vi "Read Hardware Interface Information.vi"(8 "error in (no error)":errorcluster, 10 "hardware interface index":u16, 11 "PLBB in":refnum<class "PL BlackBox Modbus Client.lvclass">) -> (0 "error out":errorcluster, 2 "hardware interface information":cluster{"type":u16, "name":string} {"type" items=["Unknown", "UART", "Network interface", "Ethernet", "Wi-Fi"]}, 3 "PLBB out":refnum<class "PL BlackBox Modbus Client.lvclass">)   [LabVIEW 2015, in "PL BlackBox Modbus Client.lvclass"]
doc: "Reads the hardware interface information."
uses:
  PL BlackBox Modbus Client.lvclass
  <vilib>/plasmapper/PL Modbus Client/PL Modbus Client.lvclass
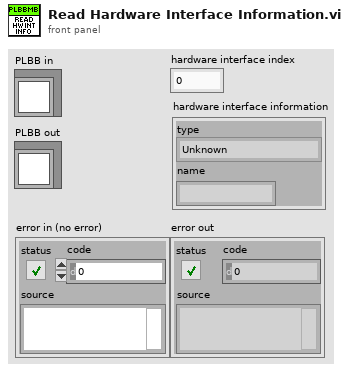
[diagram p1: front panel]
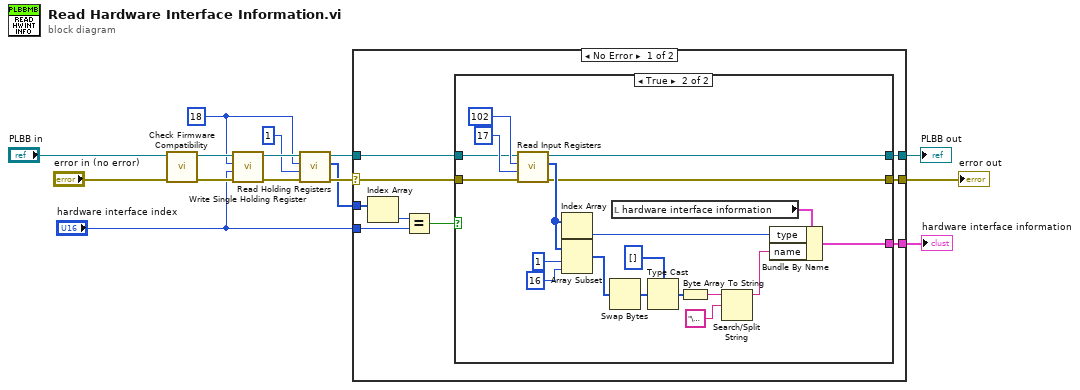
[diagram p0: block diagram]
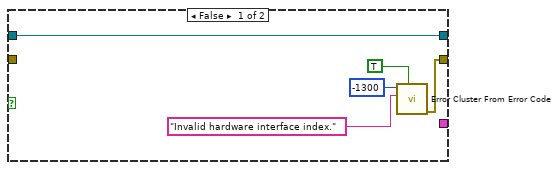
[diagram p2: hidden frame]
diagram:
  w7 = u16 18 ("address")
  n1 = call-dynamic "Check Firmware Compatibility.vi"("error in (no error)"="error in (no error)", "PLBB in"="PLBB in") -> ("error out"=w10:errorcluster, "PLBB out"=w11:refnum<class "PL BlackBox Modbus Client.lvclass">)  [unwired: 8 in]
  n2 = call <vilib>:"Write Single Holding Register.vi"("error in (no error)"=w10, "value"="hardware interface index", "address"=w7, "MODBUS in"=w11) -> ("error out"=w6:errorcluster, "MODBUS out"=w9:refnum<class "PL BlackBox Modbus Client.lvclass">)  [unwired: 6 in]
  n3 = call <vilib>:"Read Holding Registers.vi"("error in (no error)"=w6, "number of holding registers"=u16 1 ("address"), "address"=w7, "MODBUS in"=w9) -> ("error out"=w5:errorcluster, "values"=w3:u16[], "MODBUS out"=w4:refnum<class "PL BlackBox Modbus Client.lvclass">)  [unwired: 5 in]
  n4 = case shown="No Error" w5 {
    selector: w5 -> [w17 w49]
    tunnel: [w24 w49] -> w15
    tunnel: [w23 w50] -> w14
    tunnel: w4 -> [w18 w50]
    tunnel: w3 -> [w22 _]
    tunnel: "hardware interface index" -> [w20 _]
    tunnel: [w16 _] -> w1
    frame No Error {
      n5 = Index Array(array=w22) -> (element=w21:u16)  [unwired: 1 in]
      n6 = Equal?(x=w21, y=w20) -> (x = y?=w19:bool)
      n7 = case shown="True" w19 {
        tunnel: [w25 w30] -> w24
        tunnel: [w29 w31] -> w23
        tunnel: w18 -> [w29 w46]
        tunnel: w17 -> [_ w45]
        tunnel: [_ w43] -> w16
        frame False {
          n8 = call <vilib>:"Error Cluster From Error Code.vi"("show call chain? (False)"=TRUE, "error message (\"\")"="Invalid hardware interface index." ("error message (\"\")"), "error code (0)"=-1300) -> ("error out"=w25:errorcluster)  [unwired: 6 in]
        }
        frame True {
          n9 = call <vilib>:"Read Input Registers.vi"("error in (no error)"=w45, "number of input registers"=u16 17 ("address"), "address"=u16 102, "MODBUS in"=w46) -> ("error out"=w30:errorcluster, "values"=w40:u16[], "MODBUS out"=w31:refnum<class "PL BlackBox Modbus Client.lvclass">)  [unwired: 5 in]
          n10 = Index Array(array=w40) -> (element=w39:u16)  [unwired: 1 in]
          n11 = Array Subset(array=w40, index=1, length=16 ("index")) -> (w33:u16[])
          n12 = Swap Bytes(anything=w33) -> (byte swapped=w36:u16[])
          n13 = local read "hardware interface information"() -> (w44:cluster{"type":u16, "name":string})
          n14 = Type Cast(type=u8[] [] ("values"), x=w36) -> (*(type *) &x=w38:u8[])
          n15 = Byte Array To String(unsigned byte array=w38) -> (string=w35:string)
          n16 = Search/Split String(string=w35, search string/char (-)="\u0000") -> (substring before match=w32:string)  [unwired: 1 in, 2 out]
          n17 = Bundle By Name(cluster=w44, "type"=w39, "name"=w32) -> (w43:cluster{"type":u16, "name":string})
        }
      }
    }
    frame Error {
    }
  }
  "error out" <- w15
  "PLBB out" <- w14
  "hardware interface information" <- w1
